vi "Patrick-Test-Excess-64.vi"() -> ()   [LabVIEW 2019]
panel:
  out "Array 2":dbl[](array[numeric])
  out "Boolean array 2":bool[][](array[boolean])=[[FALSE, TRUE, FALSE, FALSE, FALSE, FALSE, FALSE, TRUE, FALSE, FALSE, FALSE, TRUE, FALSE, FALSE, FALSE, FALSE, FALSE, FALSE, FALSE, FALSE, FALSE, FALSE, FALSE, FALSE, FALSE, FALSE, FALSE, FALSE, FALSE, FALSE, FALSE, FALSE], [FALSE, TRUE, FALSE, FALSE, FALSE, FALSE, FALSE, TRUE, FALSE, FALSE, TRUE, FALSE, FALSE, FALSE, FALSE, FALSE, FALSE, FALSE, FALSE, FALSE, FALSE, FALSE, FALSE, FALSE, FALSE, FALSE, FALSE, FALSE, FALSE, FALSE, FALSE, FALSE], [FALSE, TRUE, FALSE, FALSE, FALSE, FALSE, FALSE, TRUE, FALSE, FALSE, TRUE, TRUE, FALSE, FALSE, FALSE, FALSE, FALSE, FALSE, FALSE, FALSE, FALSE, FALSE, FALSE, FALSE, FALSE, FALSE, FALSE, FALSE, FALSE, FALSE, FALSE, FALSE], [TRUE, TRUE, FALSE, FALSE, FALSE, FALSE, FALSE, TRUE, FALSE, FALSE, FALSE, TRUE, FALSE, FALSE, FALSE, FALSE, FALSE, FALSE, FALSE, FALSE, FALSE, FALSE, FALSE, FALSE, FALSE, FALSE, FALSE, FALSE, FALSE, FALSE, FALSE, FALSE], [TRUE, TRUE, FALSE, FALSE, FALSE, FALSE, FALSE, TRUE, FALSE, FALSE, TRUE, FALSE, FALSE, FALSE, FALSE, FALSE, FALSE, FALSE, FALSE, FALSE, FALSE, FALSE, FALSE, FALSE, FALSE, FALSE, FALSE, FALSE, FALSE, FALSE, FALSE, FALSE], [TRUE, TRUE, FALSE, FALSE, FALSE, FALSE, FALSE, TRUE, FALSE, FALSE, TRUE, TRUE, FALSE, FALSE, FALSE, FALSE, FALSE, FALSE, FALSE, FALSE, FALSE, FALSE, FALSE, FALSE, FALSE, FALSE, FALSE, FALSE, FALSE, FALSE, FALSE, FALSE], [FALSE, TRUE, TRUE, FALSE, FALSE, FALSE, FALSE, FALSE, FALSE, TRUE, FALSE, FALSE, FALSE, FALSE, FALSE, FALSE, FALSE, FALSE, FALSE, FALSE, FALSE, FALSE, FALSE, FALSE, FALSE, FALSE, FALSE, FALSE, FALSE, FALSE, FALSE, TRUE], [FALSE, FALSE, TRUE, FALSE, FALSE, FALSE, FALSE, FALSE, FALSE, TRUE, FALSE, FALSE, TRUE, TRUE, FALSE, FALSE, TRUE, TRUE, FALSE, FALSE, TRUE, TRUE, FALSE, FALSE, TRUE, TRUE, FALSE, FALSE, TRUE, TRUE, FALSE, FALSE], [FALSE, FALSE, TRUE, FALSE, FALSE, FALSE, FALSE, FALSE, FALSE, TRUE, FALSE, TRUE, TRUE, FALSE, FALSE, TRUE, TRUE, FALSE, FALSE, TRUE, TRUE, FALSE, FALSE, TRUE, TRUE, FALSE, FALSE, TRUE, TRUE, FALSE, FALSE, TRUE], [FALSE, TRUE, FALSE, FALSE, FALSE, FALSE, FALSE, TRUE, FALSE, FALSE, FALSE, TRUE, TRUE, FALSE, TRUE, TRUE, FALSE, FALSE, TRUE, TRUE, FALSE, FALSE, TRUE, TRUE, FALSE, FALSE, TRUE, TRUE, FALSE, FALSE, TRUE, TRUE], [FALSE, FALSE, FALSE, FALSE, FALSE, FALSE, FALSE, FALSE, FALSE, FALSE, FALSE, FALSE, FALSE, FALSE, FALSE, FALSE, FALSE, FALSE, FALSE, FALSE, FALSE, FALSE, FALSE, FALSE, FALSE, FALSE, FALSE, FALSE, FALSE, FALSE, FALSE, FALSE], [FALSE, TRUE, FALSE, FALSE, FALSE, FALSE, FALSE, TRUE, FALSE, FALSE, FALSE, TRUE, FALSE, FALSE, FALSE, FALSE, FALSE, FALSE, FALSE, FALSE, FALSE, FALSE, FALSE, FALSE, FALSE, FALSE, FALSE, FALSE, FALSE, FALSE, FALSE, FALSE], [FALSE, TRUE, FALSE, FALSE, FALSE, FALSE, FALSE, TRUE, TRUE, FALSE, TRUE, FALSE, FALSE, FALSE, FALSE, FALSE, FALSE, FALSE, FALSE, FALSE, FALSE, FALSE, FALSE, FALSE, FALSE, FALSE, FALSE, FALSE, FALSE, FALSE, FALSE, FALSE], [FALSE, TRUE, FALSE, FALSE, FALSE, FALSE, TRUE, FALSE, FALSE, TRUE, TRUE, FALSE, FALSE, TRUE, FALSE, FALSE, FALSE, FALSE, FALSE, FALSE, FALSE, FALSE, FALSE, FALSE, FALSE, FALSE, FALSE, FALSE, FALSE, FALSE, FALSE, FALSE], [FALSE, TRUE, FALSE, FALSE, FALSE, FALSE, TRUE, TRUE, FALSE, FALSE, TRUE, TRUE, TRUE, TRUE, TRUE, FALSE, FALSE, FALSE, FALSE, FALSE, FALSE, FALSE, FALSE, TRUE, FALSE, FALSE, FALSE, FALSE, FALSE, FALSE, FALSE, FALSE], [FALSE, TRUE, FALSE, FALSE, FALSE, TRUE, FALSE, FALSE, FALSE, FALSE, TRUE, FALSE, FALSE, TRUE, TRUE, TRUE, FALSE, FALSE, FALSE, TRUE, FALSE, FALSE, FALSE, FALSE, FALSE, FALSE, FALSE, FALSE, FALSE, FALSE, FALSE, FALSE], [FALSE, TRUE, FALSE, FALSE, FALSE, TRUE, FALSE, TRUE, FALSE, FALSE, FALSE, TRUE, TRUE, FALSE, FALSE, FALSE, FALSE, TRUE, TRUE, FALSE, TRUE, FALSE, TRUE, FALSE, FALSE, FALSE, FALSE, FALSE, FALSE, FALSE, FALSE, FALSE]]
  in  "Test numbers":u32[](array[numeric])=[1091567616, 1092616192, 1093664768, 3239051264, 3240099840, 3241148416, 1614807041, 541904076, 542742937, 1092301619, 0, 1091567616, 1101004800, 1113849856, 1128136960, 1143410688, 1159227904] format="%032b"
  out "Array":bool[][](array[boolean])=[[FALSE, FALSE, TRUE, TRUE, TRUE, TRUE, TRUE, FALSE], [FALSE, TRUE, FALSE, FALSE, FALSE, FALSE, FALSE, TRUE], [TRUE, FALSE, FALSE, FALSE, TRUE, FALSE, FALSE, TRUE], [FALSE, FALSE, TRUE, TRUE, FALSE, TRUE, TRUE, TRUE], [FALSE, TRUE, FALSE, FALSE, TRUE, FALSE, TRUE, TRUE], [TRUE, TRUE, FALSE, FALSE, FALSE, TRUE, TRUE, FALSE], [TRUE, FALSE, TRUE, FALSE, FALSE, TRUE, TRUE, TRUE], [TRUE, TRUE, TRUE, TRUE, FALSE, TRUE, FALSE, FALSE]]
  out "8 bytes":u8[](array[numeric])=[62, 65, 137, 55, 75, 198, 167, 244] format="%08b"
  out "result":dbl[](array[numeric])=[1.0, 2.0, 3.0, -1.0, -2.0, -3.0, 8.507061201264422e+37, inf, inf, 1.6999998092651367, nan, 1.0, 10.0, 100.0, 992.0625, 10000.0, 100000.0]
  # "https://boolean.klaasholwerda.nl/interface/bnf/gdsformat.html#datatypes"
  # "01000001000100000000000000000000 = 1\n01000001001000000000000000000000 = 2\n01000001001100000000000000000000 = 3\n11000001000100000000000000000000 = -1\n11000001001000000000000000000000 = -2\n11000001001100000000000000000000 = -3\n01000000100000000000000000000000 = 0 .5\n0100000010011001100110011001100 = 1 .6\n0100000010110011001100110011001 = 1 .7\n01000001000110000000000000000000 = 1.5\n01000001000110011001100110011001 = 1.6\n01000001000110110011001100110011 = 1.7\n00000000000000000000000000000000 = 0\n01000001000100000000000000000000 = 1\n01000001101000000000000000000000 = 10\n01000010011001000000000000000000 = 100\n01000011001111100000000100000000 = 1000\n01000100001001110001000000000000 = 10000\n01000101000110000110101000000000 = 100000"
  # "01000011001111100000000100000000\n01000011001111100000000100000000"
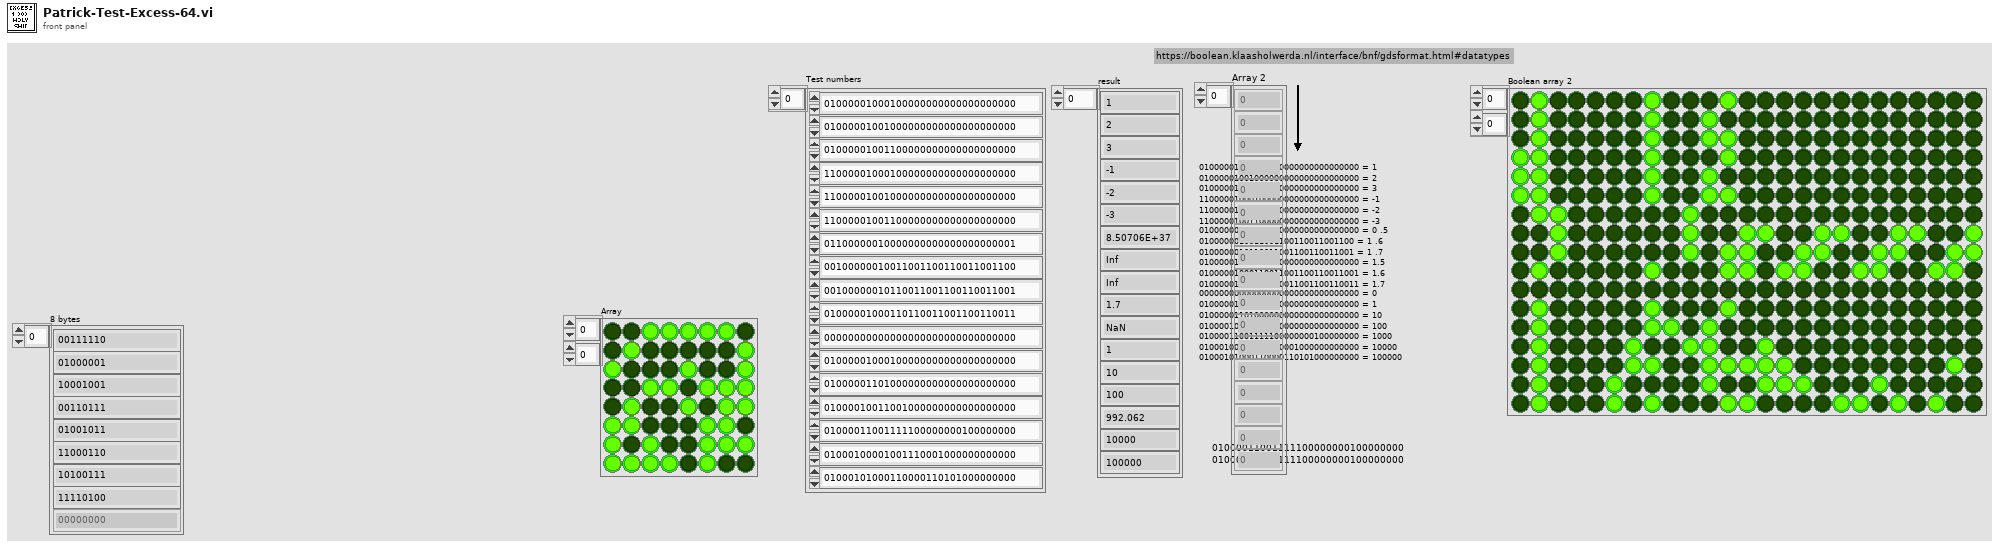
[diagram p1: front panel]
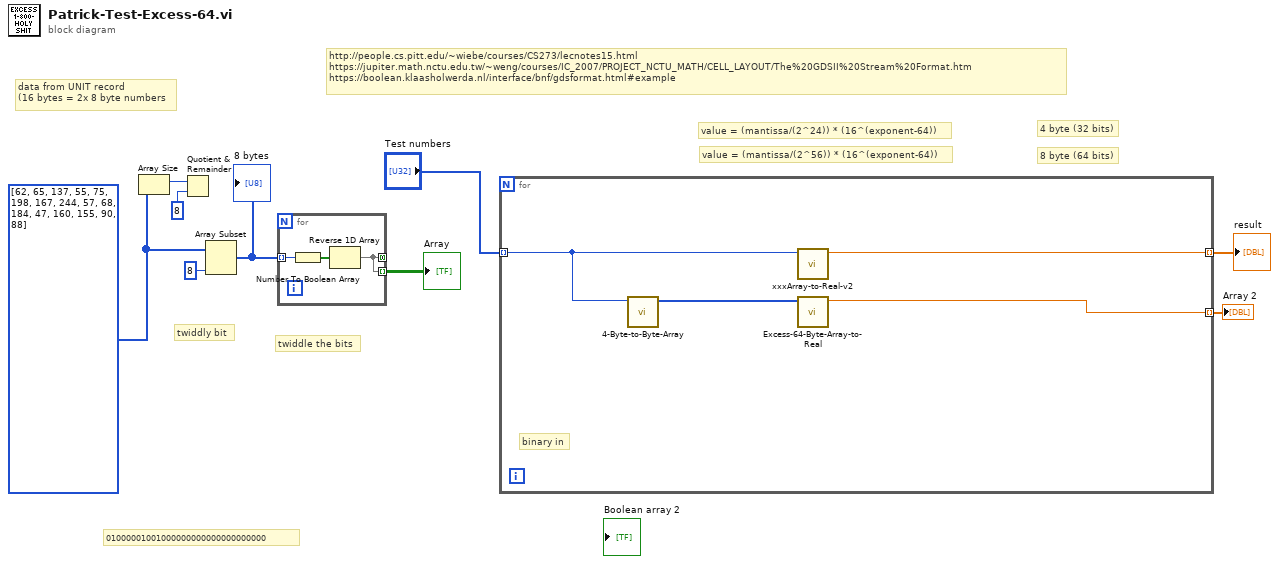
[diagram p0: block diagram]
diagram:
  w6 = u8[] [62, 65, 137, 55, 75, 198, 167, 244, 57, 68, 184, 47, 160, 155, 90, 88] ("Data")
  # "01000001001000000000000000000000"
  # "http://people.cs.pitt.edu/~wiebe/courses/CS273/lecnotes15.html\nhttps://jupiter.math.nctu.edu.tw/~weng/courses/IC_2007/PROJECT_NCTU_MATH/CELL_LAYOUT/The%20GDSII%20Stream%20Format.htm \nhttps://boolean.klaasholwerda.nl/interface/bnf/gdsformat.html#example"
  # "data from UNIT record\n(16 bytes = 2x 8 byte numbers"
  # "8 byte (64 bits)"
  # "4 byte (32 bits)"
  # "twiddly bit"
  # "twiddle the bits"
  # "value = (mantissa/(2^24)) * (16^(exponent-64))"
  # "value = (mantissa/(2^56)) * (16^(exponent-64))"
  n1 = Array Size(array=w6) -> (size(s)=w8:i32)
  n2 = Quotient & Remainder(x=w8, y=8 ("length")) -> ()  [unwired: 2 out]
  n3 = Array Subset(array=w6, length=8) -> (w4:u8[])  [unwired: 1 in]
  "8 bytes" <- w4
  n4 = for {
    tunnel: w4 -> [w12] mode=indexing
    tunnel: [w10] -> _ mode=concatenating
    tunnel: [w10] -> w3 mode=indexing
    n5 = Number To Boolean Array(number=w12) -> (Boolean array=w11:bool[])
    n6 = Reverse 1D Array(array=w11) -> (reversed array=w10:bool[])
  }
  "Array" <- w3
  n7 = for {
    tunnel: [w16] -> w7 mode=indexing
    tunnel: "Test numbers" -> [w15] mode=indexing
    tunnel: [w13] -> w1 mode=indexing
    # "binary in"
    n8 = call "4-Byte-to-Byte-Array.vi"("4 Byte in"=w15) -> ("Byte array out"=w14:u8[])  [unwired: 6 in]
    n9 = call "xxxArray-to-Real-v2.vi"("Numeric in"=w15) -> ("Numeric out"=w16:dbl)  [unwired: 10 in]
    n10 = call "Excess-64-Byte-Array-to-Real.vi"("Byte array (4 or 8 bytes)"=w14) -> ("Real Number"=w13:dbl)  [unwired: 10 in]
  }
  "result" <- w7
  "Array 2" <- w1
